vi "Arbiter.vi"(1 "Arbitration Type \n(Input)":enum16{"Sum", "Maximin"}(ring), 2 "Steps (Input)":dbl) -> (0 "Optimal Angle (Output)":dbl)   [LabVIEW 2012]
doc: "Takes in number of steps to be used, goodness functions, and arbitration type. Sends angles to gfunctions, takes weighted (based on arbitration type) sum and outputs angle from northing that is optimal."
panel:
  out "Array":dbl[](array[numeric])
  out "appended array":dbl[][](array[numeric])
  # "Arbiter: Takes in Steps, Arbitration Type, Outputs Optimal Angle"
  # "Degrees from Northing, Clockwise"
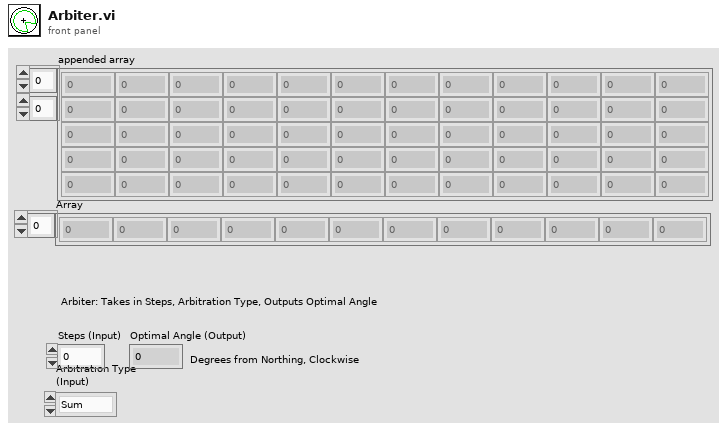
[diagram p1: front panel]
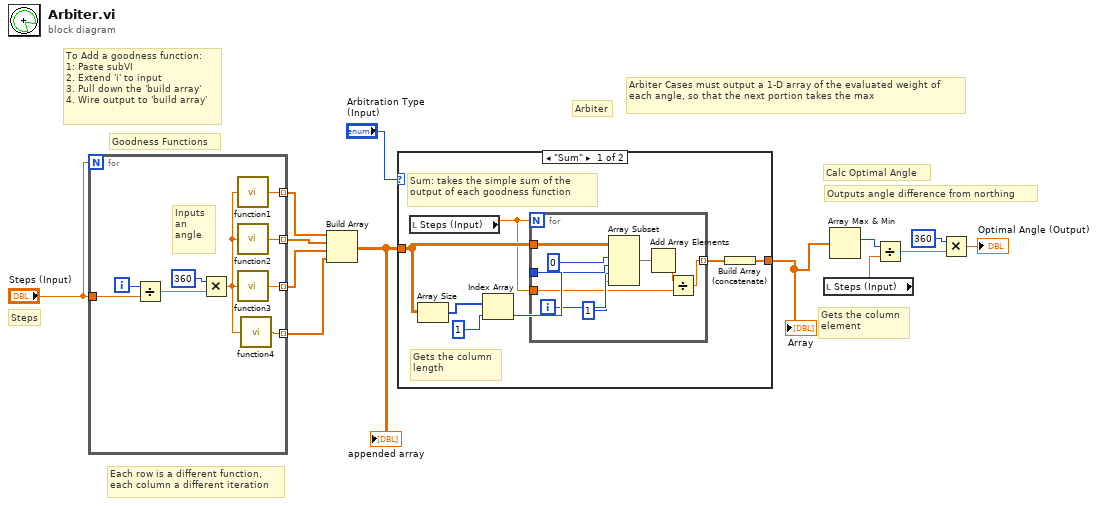
[diagram p0: block diagram]
diagram:
  # "Outputs angle difference from northing"
  # "Calc Optimal Angle"
  # "Gets the column\nelement"
  # "Arbiter Cases must output a 1-D array of the evaluated weight of each angle, so that the next portion takes the max"
  # "Arbiter"
  # "To Add a goodness function:\n1: Paste subVI\n2. Extend 'i' to input\n3. Pull down the 'build array'\n4. Wire output to 'build array'"
  # "Goodness Functions"
  # "Each row is a different function,\neach column a different iteration"
  # "Steps"
  n1 = for {
    N: "Steps (Input)" -> [_]
    tunnel: [w22] -> w11 mode=indexing
    tunnel: [w21] -> w12 mode=indexing
    tunnel: [w20] -> w13 mode=indexing
    tunnel: "Steps (Input)" -> [w18]
    tunnel: [w14] -> w1 mode=indexing
    i -> [w19]
    # "Inputs an angle"
    n2 = Divide(x=w19, y=w18) -> (x/y=w17:dbl)
    n3 = Multiply(x=360, y=w17) -> (x*y=w15:dbl)
    n4 = call "function1.vi"("y"=w15) -> ("x+y"=w22:dbl)
    n5 = call "function2.vi"("y"=w15) -> ("x+y"=w21:dbl)
    n6 = call "function3.vi"("y"=w15) -> ("x+y"=w20:dbl)
    n7 = call "function4.vi"("Input"=w15) -> ("Output"=w14:dbl)
  }
  n8 = Build Array(w11, w12, w13, w1) -> (w5:dbl[][])
  "appended array" <- w5
  n9 = case shown="\"Sum\"" "Arbitration Type \n(Input)" {
    tunnel: w5 -> [w29 _]
    tunnel: [w28 _] -> w4
    frame "Sum" {
      # "Sum: takes the simple sum of the output of each goodness function"
      # "Gets the column\nlength"
      n10 = local read "Steps (Input)"() -> (w23:dbl)
      n11 = Array Size(array=w29) -> (size(s)=w27:i32[])
      n12 = Index Array(array=w27, index=1) -> (element=w25:i32)
      n13 = for {
        N: w23 -> [_]
        tunnel: w29 -> [w38]
        tunnel: [w31] -> w24 mode=indexing
        tunnel: w25 -> [w35]
        tunnel: w23 -> [w30]
        i -> [w34]
        n14 = Array Subset(array=w38, index (row)=0, length (row)=w35, index (col)=w34, length (col)=1) -> (w37:dbl[][])
        n15 = Add Array Elements(numeric array=w37) -> (sum=w32:dbl)
        n16 = Divide(x=w32, y=w30) -> (x/y=w31:dbl)
      }
      n17 = Build Array (concatenate)(w24) -> (w28:dbl[])
    }
    frame "Maximin" {
    }
  }
  "Array" <- w4
  n18 = local read "Steps (Input)"() -> (w6:dbl)
  n19 = Array Max & Min(array=w4) -> (max index (indices)=w2:i32)  [unwired: 3 out]
  n20 = Divide(x=w2, y=w6) -> (x/y=w7:dbl)
  n21 = Multiply(x=360, y=w7) -> (x*y=→"Optimal Angle (Output)":dbl)
